vi "RT 1.0.vi"() -> ()   [LabVIEW 2014]
uses:
  <vilib>/FPGAPlugInAG/myRIO-1950/niLvFpga_Open_myRIO-1950.vi
  <vilib>/rvi/interface/common/dynamic/niFpgaDynamicAddResources.vi
  <vilib>/Utility/error.llb/Error Cluster From Error Code.vi
  <vilib>/rvi/errors/niLvFpgaAdjustHostInterfaceError.vi
  <vilib>/FPGAPlugInAG/Dynamic/niLvFpga_Close_Dynamic.vi
  <vilib>/rvi/interface/nirviOpenFPGA/nirviOpenFPGA.xnode
  FPGA Bitfiles/SensorMain_FPGATarget_ParallaxPING)))(_3ylNEQ+tG2M.lvbitx
  <instrlib>/Parallax PING)))/FPGA Example/Parallax PING))) (FPGA).vi
  <vilib>/rvi/interface/nirviReadWriteControl/nirviReadWriteControl.xnode
  <vilib>/rvi/interface/nirviCloseFPGA/nirviCloseFPGA.xnode
  NiFpgaLv.dll
  <vilib>/rvi/interface/Simulation/niFpgaSimulationCallBeginRW.vi
panel:
  in  "Tab Control":enum32{"Page 1", "Page 2"}(tab)
  in  "stop":bool
  out "Front":fxp<+,64,16>
  out "Front Side":fxp<+,64,16>
  out "Back Side":fxp<+,64,16>
  out "Back":fxp<+,32,8>
  out "Time Elapsed":u32
  out "Left Radio":bool
  out "Right Radio":bool
  out "State":T1(ring)
  out "myRio / RC Control":bool
  out "Backward Radio":bool
  out "Forward Radio":bool
  in  "Left/Right Speed":u32
  in  "Left/Right":enum16{"Left", "Right", "Stop"}(ring)
  in  "Front/Back Speed":u32
  in  "Front/Back":enum16{"Forward", "Backward", "Stop"}(ring)
  out "State RT":T2(ring)
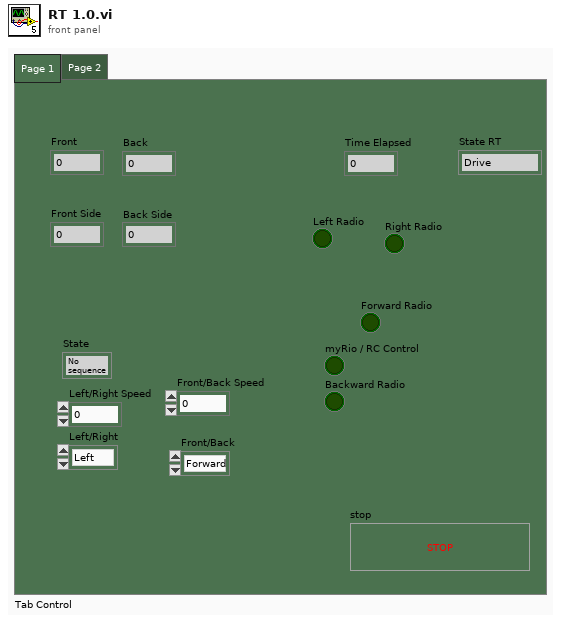
[diagram p1: front panel]
types:
  T1 = enum16{"No sequence", "Right 1", "Left 1", "Right 2", "Left 2"}
  T2 = enum16{"Drive", "Pre Start 1", "Pre Start 2", "Start", "Middle", "Back Up", "Turn In", "Back In", "Straight", "End"}
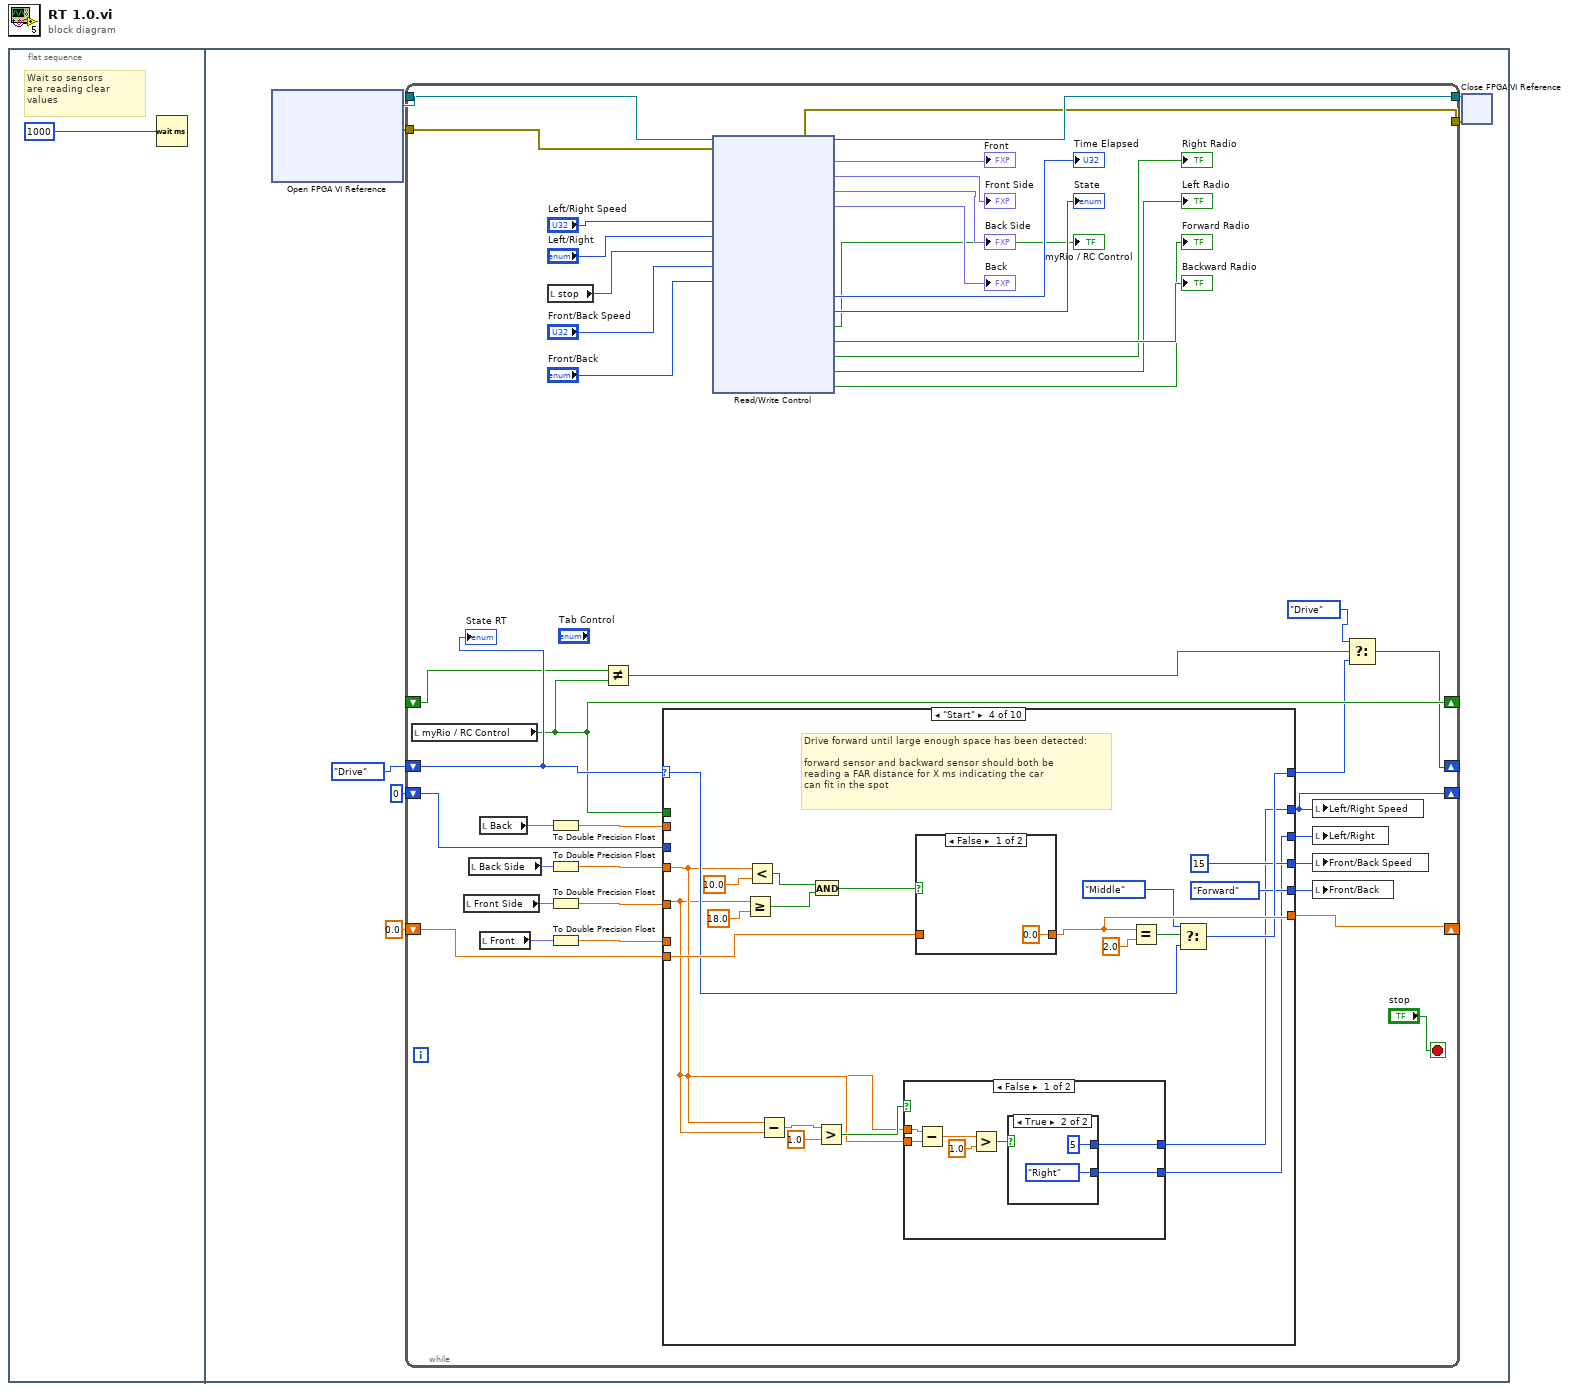
[diagram p0: block diagram]
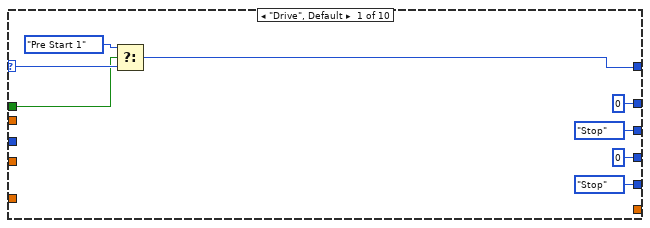
[diagram p2: hidden frame]
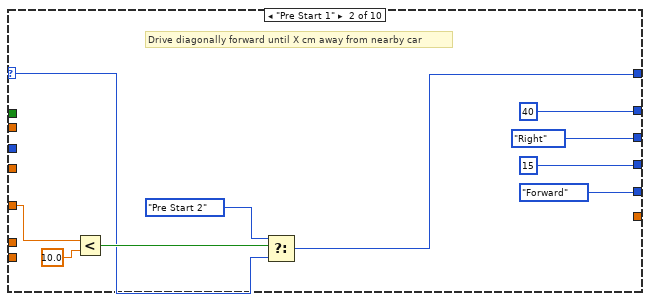
[diagram p3: hidden frame]
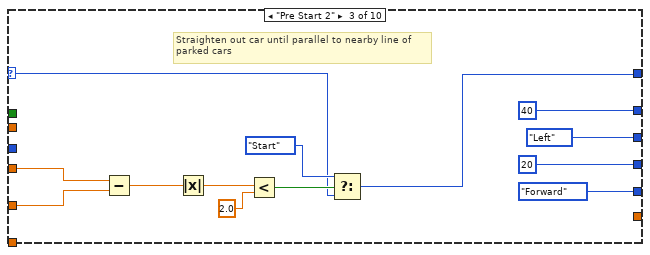
[diagram p4: hidden frame]
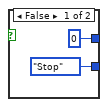
[diagram p5: hidden frame]
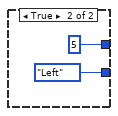
[diagram p6: hidden frame]
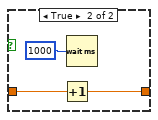
[diagram p7: hidden frame]
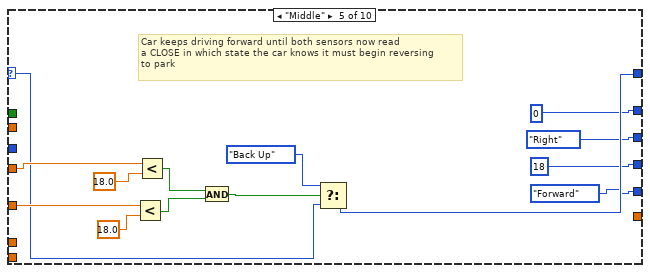
[diagram p8: hidden frame]
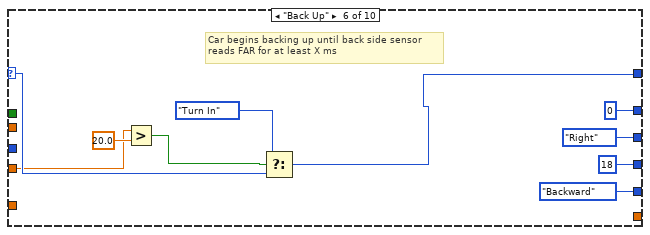
[diagram p9: hidden frame]
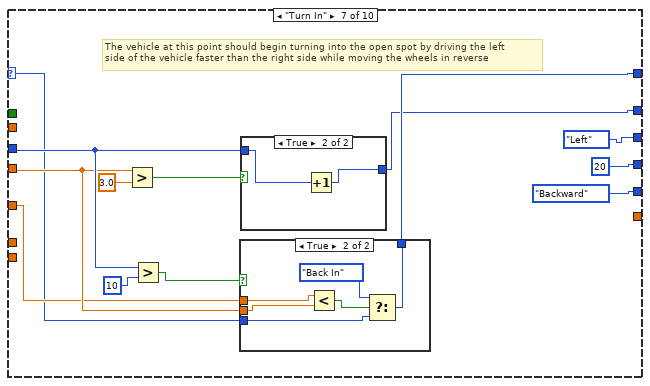
[diagram p10: hidden frame]
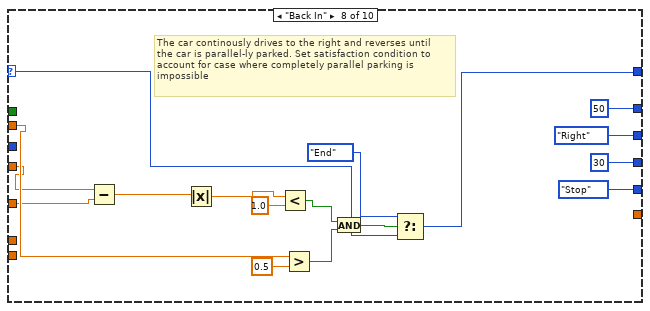
[diagram p13: hidden frame]
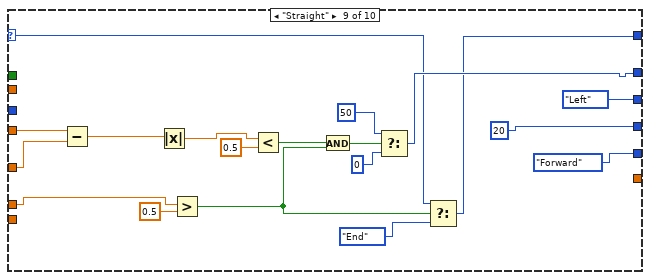
[diagram p14: hidden frame]
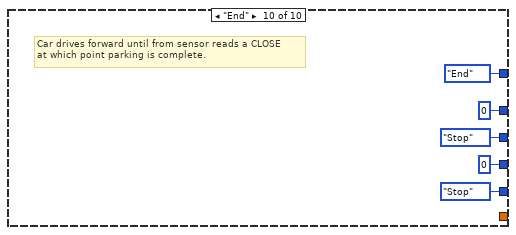
[diagram p15: hidden frame]
diagram:
  n1 = flat-sequence {
    frame #0 {
      # "Wait so sensors\nare reading clear\nvalues"
      n2 = Wait (ms)(milliseconds to wait=u32 1000) -> ()  [unwired: 1 out]
    }
    frame #1 {
      n3 = xnode "Open FPGA VI Reference"() -> ("FPGA VI Reference Out"=w7:refnum<k20>, "error out"=w5:errorcluster)  [unwired: 2 in]
      n4 = while {
        shift-right: [w9] -> _
        shift-left: T2."Drive" -> [w50]
        tunnel: w7 -> [w49]
        tunnel: [w48] -> w6
        tunnel: w5 -> [w47]
        tunnel: [w46] -> w4
        shift-right: [w17] -> _
        shift-left: 0.0 -> [w18]
        shift-right: [w16] -> _
        shift-left: u32 0 ("Left/Right Speed") -> [w15]
        shift-right: [w13] -> _
        shift-left: _ -> [w14]
        stop <- "stop" stop-if-true
        n5 = local read "myRio / RC Control"() -> (w13:bool)
        n6 = local read "Front Side"() -> (w23:fxp<+,64,16>)
        n7 = local read "Back Side"() -> (w25:fxp<+,64,16>)
        n8 = local read "Back"() -> (w26:fxp<+,32,8>)
        n9 = local read "Front"() -> (w22:fxp<+,64,16>)
        n10 = local read "stop"() -> (w39:bool)
        n11 = To Double Precision Float(number=w26) -> (double precision float=w19:dbl)
        n12 = To Double Precision Float(number=w25) -> (double precision float=w24:dbl)
        n13 = To Double Precision Float(number=w23) -> (double precision float=w20:dbl)
        n14 = To Double Precision Float(number=w22) -> (double precision float=w21:dbl)
        n15 = Not Equal?(x=w14, y=w13) -> (x != y?=w12:bool)
        n16 = case shown="\"Start\"" w50 {
          selector: w50 -> [w59 w62 w71 w93 w126 w137 w148 w172 w185 _]
          tunnel: [w57 w63 w70 w92 w125 w136 w153 w171 w186 T2."End" ("t")] -> w10
          tunnel: w13 -> [w56 _ _ _ _ _ _ _ _ _]
          tunnel: [enum16{"Left", "Right", "Stop"}."Stop" ("Left/Right") enum16{"Left", "Right", "Stop"}."Right" ("Left/Right") enum16{"Left", "Right", "Stop"}."Left" ("Left/Right") w85 enum16{"Left", "Right", "Stop"}."Right" ("Left/Right") enum16{"Left", "Right", "Stop"}."Right" ("Left/Right") enum16{"Left", "Right", "Stop"}."Left" ("Left/Right") enum16{"Left", "Right", "Stop"}."Right" ("Left/Right") enum16{"Left", "Right", "Stop"}."Left" ("Left/Right") enum16{"Left", "Right", "Stop"}."Stop" ("Left/Right")] -> w29
          tunnel: [u32 0 ("f") u32 40 ("Left/Right Speed") u32 40 ("Left/Right Speed") w86 u32 0 ("Left/Right Speed") u32 0 ("Left/Right Speed") w151 u32 50 ("Left/Right Speed") w191 u32 0 ("f")] -> w16
          tunnel: [u32 0 ("Front/Back Speed") u32 15 ("Front/Back Speed") u32 20 ("Front/Back Speed") u32 15 ("Front/Back Speed") u32 18 ("Front/Back Speed") u32 18 ("Front/Back Speed") u32 20 ("Front/Back Speed") u32 30 ("Front/Back Speed") u32 20 ("Front/Back Speed") u32 0 ("Front/Back Speed")] -> w28
          tunnel: [enum16{"Forward", "Backward", "Stop"}."Stop" ("Front/Back") enum16{"Forward", "Backward", "Stop"}."Forward" ("Front/Back") enum16{"Forward", "Backward", "Stop"}."Forward" ("Front/Back") enum16{"Forward", "Backward", "Stop"}."Forward" ("Front/Back") enum16{"Forward", "Backward", "Stop"}."Forward" ("Front/Back") enum16{"Forward", "Backward", "Stop"}."Backward" ("Front/Back") enum16{"Forward", "Backward", "Stop"}."Backward" ("Front/Back") enum16{"Forward", "Backward", "Stop"}."Stop" ("Front/Back") enum16{"Forward", "Backward", "Stop"}."Forward" ("Front/Back") enum16{"Forward", "Backward", "Stop"}."Stop" ("Front/Back")] -> w27
          tunnel: w21 -> [_ _ _ _ _ _ _ _ w192 _]
          tunnel: w24 -> [_ _ w78 w84 w131 w135 w150 w169 w194 _]
          tunnel: w20 -> [_ w60 w77 w83 w130 _ w149 w168 w193 _]
          tunnel: w19 -> [_ _ _ _ _ _ _ w170 _ _]
          tunnel: w18 -> [_ _ _ w98 _ _ _ _ _ _]
          tunnel: [_ _ _ w95 _ _ _ _ _ _] -> w17
          tunnel: w15 -> [_ _ _ _ _ _ w152 _ _ _]
          frame "Drive", Default {
            n17 = Select(t=T2."Pre Start 1", s=w56, f=w59) -> (s? t:f=w57:T2)
          }
          frame "Pre Start 1" {
            # "Drive diagonally forward until X cm away from nearby car"
            n18 = Less?(x=w60, y=10.0) -> (x < y?=w65:bool)
            n19 = Select(t=T2."Pre Start 2", s=w65, f=w62) -> (s? t:f=w63:T2)
          }
          frame "Pre Start 2" {
            # "Straighten out car until parallel to nearby line of \nparked cars"
            n20 = Subtract(x=w78, y=w77) -> (x-y=w76:dbl)
            n21 = Absolute Value(x=w76) -> (abs(x)=w75:dbl)
            n22 = Less?(x=w75, y=2.0) -> (x < y?=w73:bool)
            n23 = Select(t=T2."Start", s=w73, f=w71) -> (s? t:f=w70:T2)
          }
          frame "Start" {
            # "Drive forward until large enough space has been detected:\n\nforward sensor and backward sensor should both be \nreading a FAR distance for X ms indicating the car \ncan fit in the spot"
            n24 = Greater Or Equal?(x=w83, y=18.0) -> (x >= y?=w100:bool)
            n25 = Less?(x=w84, y=10.0) -> (x < y?=w101:bool)
            n26 = Subtract(x=w84, y=w83) -> (x-y=w89:dbl)
            n27 = And(x=w101, y=w100) -> (x .and. y?=w99:bool)
            n28 = Greater?(x=w89, y=1.0) -> (0:w87:bool)
            n29 = case shown="False" w87 {
              tunnel: [w104 u32 5 ("Left/Right Speed")] -> w86
              tunnel: [w105 enum16{"Left", "Right", "Stop"}."Left" ("Left/Right")] -> w85
              tunnel: w84 -> [w108 _]
              tunnel: w83 -> [w107 _]
              frame False {
                n30 = Subtract(x=w107, y=w108) -> (x-y=w109:dbl)
                n31 = Greater?(x=w109, y=1.0) -> (0:w106:bool)
                n32 = case shown="True" w106 {
                  tunnel: [enum16{"Left", "Right", "Stop"}."Stop" ("Left/Right") enum16{"Left", "Right", "Stop"}."Right" ("Left/Right")] -> w105
                  tunnel: [u32 0 ("Left/Right Speed") u32 5 ("Left/Right Speed")] -> w104
                  frame False {
                  }
                  frame True {
                  }
                }
              }
              frame True {
              }
            }
            n33 = case shown="False" w99 {
              tunnel: [0.0 w119] -> w95
              tunnel: w98 -> [_ w118]
              frame False {
              }
              frame True {
                n34 = Increment(x=w118) -> (x+1=w119:dbl)
                n35 = Wait (ms)(milliseconds to wait=u32 1000) -> ()  [unwired: 1 out]
              }
            }
            n36 = Equal?(x=w95, y=2.0) -> (x = y?=w96:bool)
            n37 = Select(t=T2."Middle", s=w96, f=w93) -> (s? t:f=w92:T2)
          }
          frame "Middle" {
            # "Car keeps driving forward until both sensors now read\na CLOSE in which state the car knows it must begin reversing\nto park"
            n38 = Less?(x=w130, y=18.0) -> (x < y?=w134:bool)
            n39 = Less?(x=w131, y=18.0) -> (x < y?=w133:bool)
            n40 = And(x=w133, y=w134) -> (x .and. y?=w128:bool)
            n41 = Select(t=T2."Back Up", s=w128, f=w126) -> (s? t:f=w125:T2)
          }
          frame "Back Up" {
            # "Car begins backing up until back side sensor\nreads FAR for at least X ms"
            n42 = Greater?(x=w135, y=20.0) -> (0:w139:bool)
            n43 = Select(t=T2."Turn In", s=w139, f=w137) -> (s? t:f=w136:T2)
          }
          frame "Turn In" {
            # "The vehicle at this point should begin turning into the open spot by driving the left\nside of the vehicle faster than the right side while moving the wheels in reverse"
            n44 = Greater?(x=w150, y=3.0) -> (0:w156:bool)
            n45 = Greater?(x=w152, y=u32 10) -> (0:w154:bool)
            n46 = case shown="True" w154 {
              tunnel: w149 -> [_ w164]
              tunnel: w150 -> [_ w163]
              tunnel: w148 -> [w158 w160]
              tunnel: [w158 w159] -> w153
              frame False {
              }
              frame True {
                n47 = Less?(x=w164, y=w163) -> (x < y?=w162:bool)
                n48 = Select(t=T2."Back In", s=w162, f=w160) -> (s? t:f=w159:T2)
              }
            }
            n49 = case shown="True" w156 {
              tunnel: w152 -> [w165 w167]
              tunnel: [w165 w166] -> w151
              frame False {
              }
              frame True {
                n50 = Increment(x=w167) -> (x+1=w166:u32)
              }
            }
          }
          frame "Back In" {
            # "The car continously drives to the right and reverses until\nthe car is parallel-ly parked. Set satisfaction condition to \naccount for case where completely parallel parking is \nimpossible"
            n51 = Subtract(x=w169, y=w168) -> (x-y=w184:dbl)
            n52 = Absolute Value(x=w184) -> (abs(x)=w183:dbl)
            n53 = Less?(x=w183, y=1.0) -> (x < y?=w178:bool)
            n54 = Greater?(x=w170, y=0.5) -> (0:w179:bool)
            n55 = And(x=w178, y=w179) -> (x .and. y?=w177:bool)
            n56 = Select(t=T2."End", s=w177, f=w172) -> (s? t:f=w171:T2)
          }
          frame "Straight" {
            n57 = Subtract(x=w194, y=w193) -> (x-y=w202:dbl)
            n58 = Absolute Value(x=w202) -> (abs(x)=w201:dbl)
            n59 = Greater?(x=w192, y=0.5) -> (0:w199:bool)
            n60 = Less?(x=w201, y=0.5) -> (x < y?=w198:bool)
            n61 = And(x=w198, y=w199) -> (x .and. y?=w197:bool)
            n62 = Select(t=u32 50 ("Left/Right Speed"), s=w197, f=u32 0) -> (s? t:f=w191:u32)
            n63 = Select(t=w185, s=w199, f=T2."End") -> (s? t:f=w186:T2)
          }
          frame "End" {
            # "Car drives forward until from sensor reads a CLOSE\nat which point parking is complete."
          }
        }
        n64 = xnode "Read/Write Control"("FPGA VI Reference In"=w49, "error in"=w47, "Left/Right Speed"="Left/Right Speed", "Left/Right"="Left/Right", "STOP"=w39, "Front/Back Speed"="Front/Back Speed", "Front/Back 2"="Front/Back") -> ("FPGA VI Reference Out"=w48:refnum<k20>, "error out"=w46:errorcluster, "Front"=→"Front":fxp<+,64,16>, "Left"=→"Front Side":fxp<+,64,16>, "Right"=→"Back Side":fxp<+,64,16>, "Back"=→"Back":fxp<+,32,8>, "Time Elapsed"=→"Time Elapsed":u32, "State"=→"State":T1, "myRio / RC Control"=→"myRio / RC Control":bool, "Backward Radio"=→"Backward Radio":bool, "Right Radio"=→"Right Radio":bool, "Left Radio"=→"Left Radio":bool, "Forward Radio"=→"Forward Radio":bool)
        n65 = local write "Left/Right Speed"(w16) -> ()
        n66 = local write "Left/Right"(w29) -> ()
        n67 = local write "Front/Back Speed"(w28) -> ()
        n68 = local write "Front/Back"(w27) -> ()
        n69 = Select(t=T2."Drive", s=w12, f=w10) -> (s? t:f=w9:T2)
        "State RT" <- w50
      }
      n70 = xnode "Close FPGA VI Reference"("FPGA VI Reference In"=w6, "error in"=w4) -> ()  [unwired: 1 out]
    }
  }
